vi "Variable@LPop__Parameter.vi"(1 "ParamterIn":string) -> (0 "ParamterOut":string)   [LabVIEW 2020]
panel:
  in  "Section":string(combo)
  in  "ParameterName":string(combo)
  in  "Confirm":bool
  # "Variable@LPop $Variable(,$Section)"
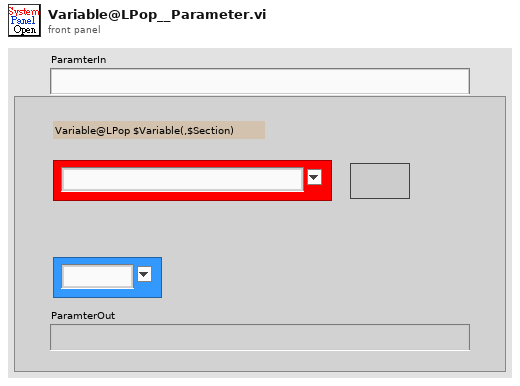
[diagram p1: front panel]
types:
  T1 = enum16{"Get", "Init", "Set", "Delete", "GetElement", "Inc", "Dec", "ReName"}
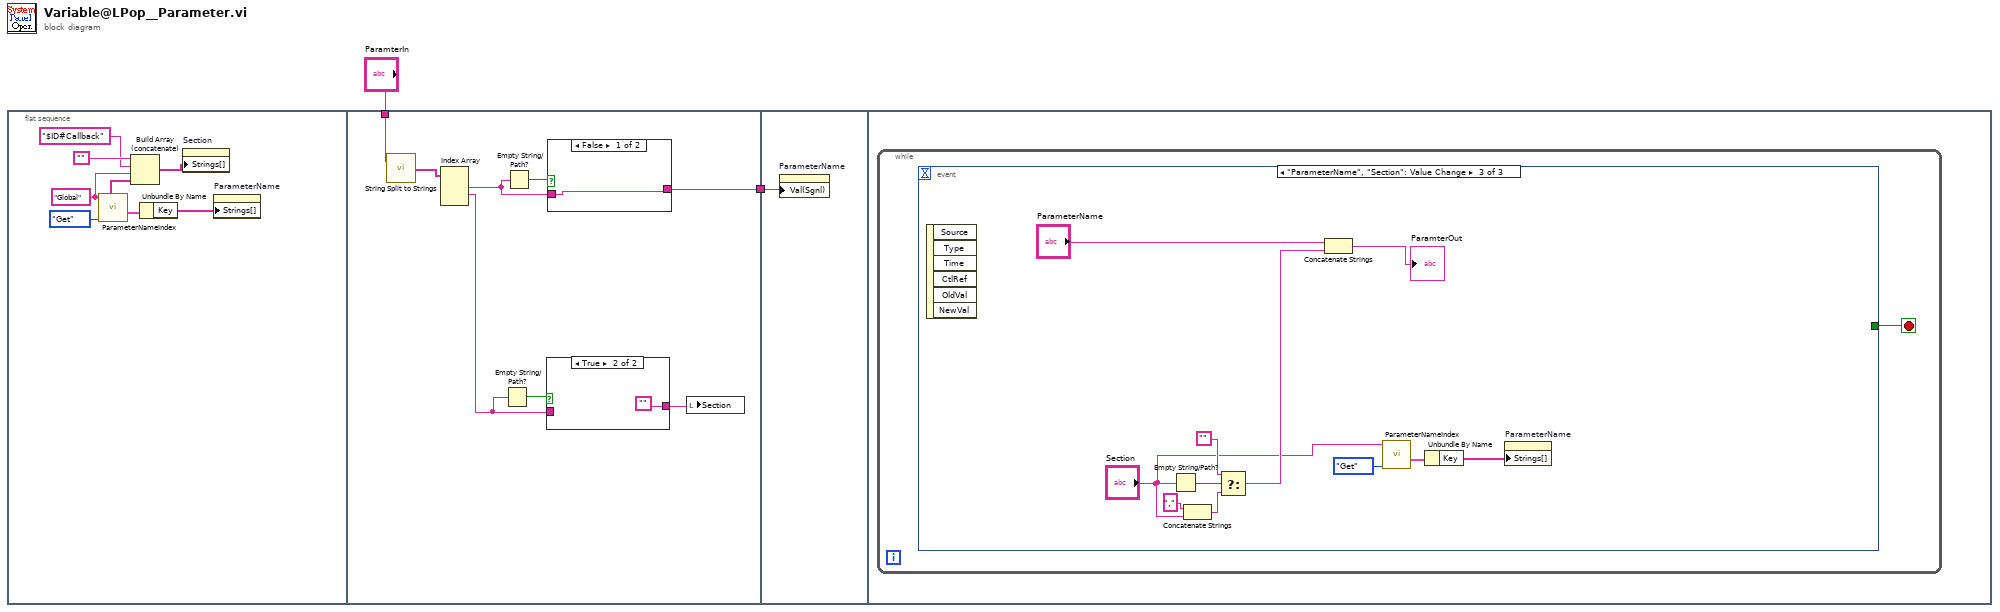
[diagram p0: block diagram]
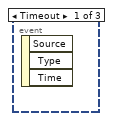
[diagram p4: hidden frame]
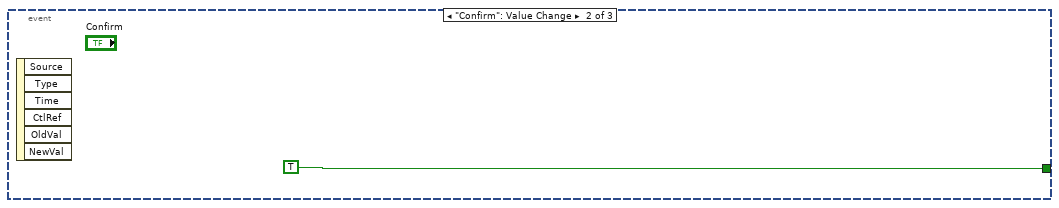
[diagram p5: hidden frame]
diagram:
  n1 = flat-sequence {
    tunnel: "ParamterIn" -> [w16]
    tunnel: [w17] -> w1
    tunnel: w1 -> [w23]
    frame #0 {
      w5 = "Global" ("VariableSection")
      n2 = call "ParameterNameIndex.vi"("OP"=T1."Get", "VariableSection"=w5) -> ("GlobalKeyValue"=w10:cluster{"Key":string[], "Value":string[]}, "SectionList"=w6:string[])  [unwired: 3 in, 5 out]
      n3 = Build Array (concatenate)("", "$ID#Callback" ("VariableSection"), w5, w6) -> (w4:string[])
      n4 = Unbundle By Name(w10) -> ("Key"=w9:string[])
      n5 = property on="Section" class="CmbBox"("Strings[]"=w4) -> ()  [unwired: 2 in, 2 out]
      n6 = property on="ParameterName" class="CmbBox"("Strings[]"=w9) -> ()  [unwired: 2 in, 2 out]
    }
    frame #1 {
      n7 = call "String Split to Strings.vi"("String"=w16) -> ("Array"=w15:string[])  [unwired: 1 in]
      n8 = Index Array(array=w15) -> (element #1=w14:string, element #2=w11:string)  [unwired: 3 in, 1 out]
      n9 = Empty String/Path?(string/path=w11) -> (empty?=w13:bool)
      n10 = Empty String/Path?(string/path=w14) -> (empty?=w18:bool)
      n11 = case shown="True" w13 {
        tunnel: w11 -> [w19 _]
        tunnel: [w19 ""] -> w12
        frame False {
        }
        frame True {
        }
      }
      n12 = case shown="False" w18 {
        tunnel: w14 -> [w21 w22]
        tunnel: [w21 w22] -> w17
        frame False {
        }
        frame True {
        }
      }
      n13 = local write "Section"(w12) -> ()
    }
    frame #2 {
      n14 = property on="ParameterName" class="CmbBox"("Val(Sgnl)"=w23) -> ()  [unwired: 2 in, 2 out]
    }
    frame #3 {
      n15 = while {
        stop <- w24 stop-if-true
        n16 = event shown="[2] \"ParameterName\", \"Section\": Value Change" {
          selector: _ -> [_ _ _]
          dyn-events: _ -> [_ _ _]
          timeout: _ -> [_ _ _]
          tunnel: [_ TRUE _] -> w24
          event Timeout {
            n17 = event-data() -> ()  [unwired: 1 in, 3 out]
          }
          event "Confirm": Value Change {
            n18 = event-data() -> ()  [unwired: 1 in, 6 out]
          }
          event "ParameterName", "Section": Value Change {
            n19 = event-data() -> ()  [unwired: 1 in, 6 out]
            n20 = Empty String/Path?(string/path="Section") -> (empty?=w32:bool)
            n21 = Concatenate Strings("," ("string"), "Section") -> (w33:string)
            n22 = Select(t="", s=w32, f=w33) -> (s? t:f=w29:string)
            n23 = Concatenate Strings("ParameterName", w29) -> (→"ParamterOut":string)
            n24 = call "ParameterNameIndex.vi"("OP"=T1."Get", "VariableSection"="Section") -> ("GlobalKeyValue"=w27:cluster{"Key":string[], "Value":string[]})  [unwired: 3 in, 6 out]
            n25 = Unbundle By Name(w27) -> ("Key"=w31:string[])
            n26 = property on="ParameterName" class="CmbBox"("Strings[]"=w31) -> ()  [unwired: 2 in, 2 out]
          }
        }
      }
    }
  }
